vi "fromWinId.vi"(8 "Error In":errorcluster, 10 "id":u64) -> (0 "Error Out":errorcluster, 2 "Value":refnum<class "QWindow.lvclass">)   [LabVIEW 2014, in "QWindow.lvclass"]
doc: "LabVIEW-specific documentation is not yet available. See <b>https://doc.qt.io/qt-5/qwindow.html#fromWinId</b>"
uses:
  QWindow.lvclass
  LQ Core/LQ Core.lvlib
  LQ Core/LQCoreEngine/LQCoreEngine.lvclass
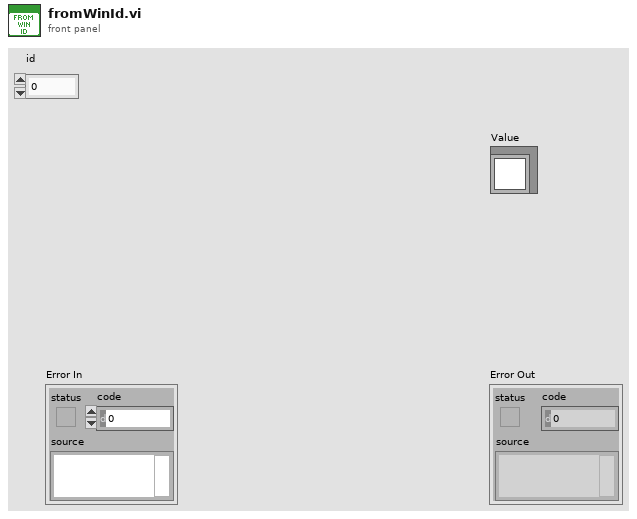
[diagram p1: front panel]
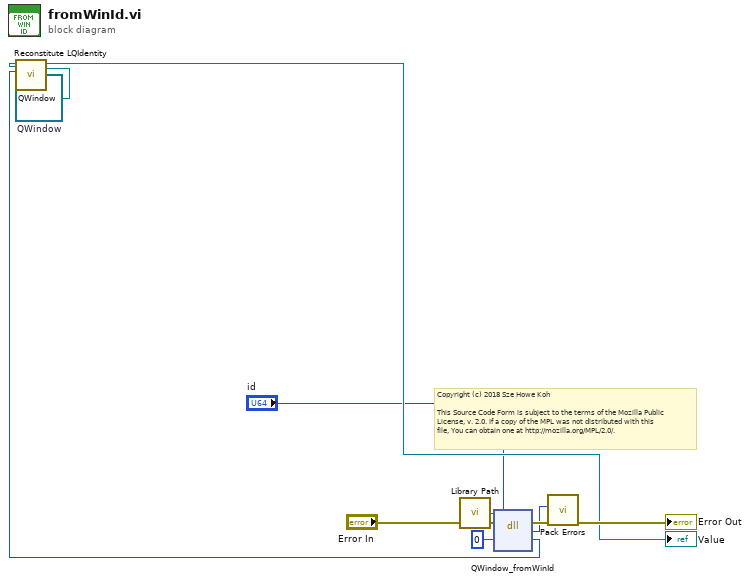
[diagram p0: block diagram]
diagram:
  w2 = refnum<class "QWindow.lvclass"> refnum  # QWindow
  # "Copyright (c) 2018 Sze Howe Koh\n\nThis Source Code Form is subject to the terms of the Mozilla Public\nLicense, v. 2.0. If a copy of the MPL was not distributed with this\nfile, You can obtain one at http://mozilla.org/MPL/2.0/."
  n1 = call "Library Path.vi"() -> ("Library Path"=w9:path)
  n2 = dll-call lib="?" fn="QWindow_fromWinId"(path in=w9, error in="Error In", "_retVal"=u64 0 ("retVal"), "id"="id") -> (error out=w7:errorcluster, w5:i32, "_retVal"=w3:u64)  [unwired: 2 in, 1 out]
  n3 = call "Reconstitute LQIdentity.vi"("Manifestation"=w3, "LQIdentity Prototype"=w2) -> ("Reconstituted LQIdentity"=→"Value":refnum<class "QWindow.lvclass">)  [unwired: 8 in, 1 out]
  n4 = call "Pack Errors.vi"("Error In"=w7, "Error Code"=w5) -> ("Error Out"=→"Error Out":errorcluster)  [unwired: 9 in]
